vi "V7310.RTC.Get.vi"(6 "timeout ms (5000)":i32=5000, 8 "error in":errorcluster, 11 "Connection in":refnum<k5>) -> (0 "error out":errorcluster, 1 "RTC string":string, 2 "RTC":timestamp, 3 "Connection out":refnum<k5>)   [LabVIEW 2016]
uses:
  LowLevel/V7310.Commands.ctl
  <vilib>/Utility/miscctls.llb/LVDateTimeRec.ctl
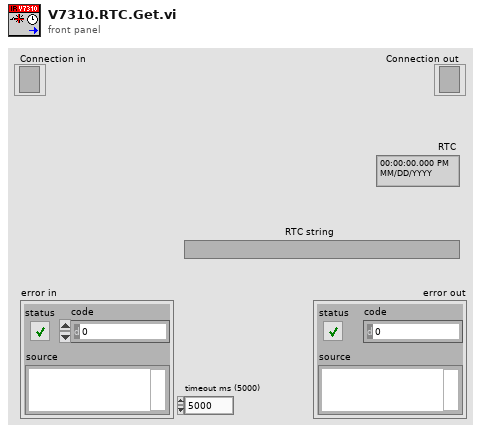
[diagram p1: front panel]
types:
  T1 = typedef "LVDateTimeRec.ctl" = cluster{"fractional second":dbl, "second":i32, "minute":i32, "hour":i32, "day of month":i32, "month":i32, "year":i32, "day of week":i32, "day of year":i32, "DST":i32}
  T2 = typedef "V7310.Commands.ctl" = enum16{"Start", "Stop", "GetStatus", "GetVarNames", "GetJobNames", "SetJob", "GetJob", "SetVars", "GetVars", "SetLayoutPosition", "SetRotation", "GetMessageID", "GetMessages", "ConfirmMessages", "DeleteMessages", "SetRTC", "GetRTC", "SetVarPosition", "SetIntensity", "GetIntensity", "SetStartTriggerDelay", "GetStartTriggerDelay", "SetStopTriggerDelay", "GetStopTriggerDelay", "SetConsecutiveTriggerDelay", "GetConsecutiveTriggerDelay", "SetMarkSpeed", "GetMarkSpeed"}
  T3 = typedef "V7310.ErrorLevels.ctl" = enum16{"OK", "Warning", "Error"}
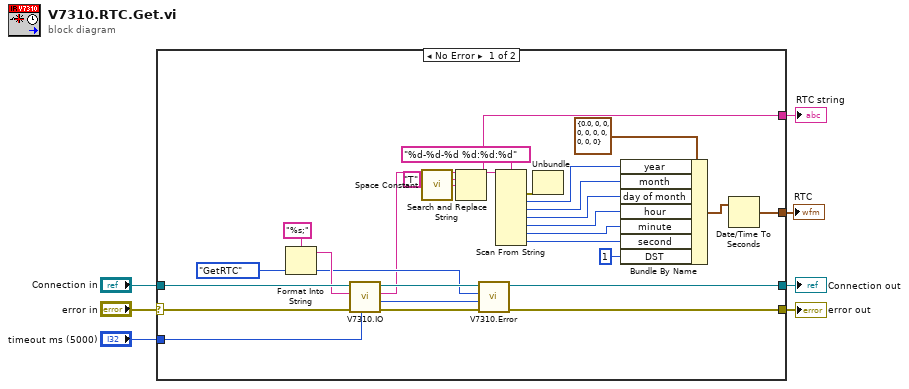
[diagram p0: block diagram]
diagram:
  n1 = case shown="No Error" "error in" {
    selector: "error in" -> [w31 w34]
    tunnel: "Connection in" -> [w32 w35]
    tunnel: [w33 w35] -> w6
    tunnel: "timeout ms (5000)" -> [w30 _]
    tunnel: [w24 w34] -> w3
    tunnel: [w23 _] -> w2
    tunnel: [w10 _] -> w1
    frame No Error {
      w27 = V7310.Commands."GetRTC" ("Cmd")
      n2 = Format Into String(format string="%s;", w27) -> (resulting string=w28:string)  [unwired: 2 in, 1 out]
      n3 = call "V7310.IO.vi"("timeout ms (5000)"=w30, "error in"=w31, "Data in"=w28, "Connection in"=w32) -> ("error out"=w25:errorcluster, "Error Level"=w26:T3, "Data out"=w20:string, "Connection out"=w33:refnum<k5>)  [unwired: 4 in]
      n4 = call <vilib>:"Space Constant.vi"() -> ("String"=w22:string)
      n5 = Search and Replace String(input string=w20, search string="T", replace string=w22) -> (result string=w10:string)  [unwired: 5 in, 3 out]
      n6 = call "V7310.Error.vi"("error in"=w25, "Error Level"=w26, "Cmd"=w27) -> ("error out"=w24:errorcluster)  [unwired: 8 in]
      n7 = Scan From String(format string="%d-%d-%d %d:%d:%d", input string=w10) -> (error out=w9:errorcluster, output 1=w17:i32, output 2=w16:i32, output 3=w15:i32, output 4=w14:i32, output 5=w13:i32, output 6=w12:i32)  [unwired: 8 in, 2 out]
      n8 = Unbundle(w9) -> ()  [unwired: 3 out]
      n9 = Bundle By Name(cluster=T1 {"fractional second"=0.0, "second"=0, "minute"=0, "hour"=0, "day of month"=0, "month"=0, "year"=0, "day of week"=0, "day of year"=0, "DST"=0} ("date time rec"), "year"=w17, "month"=w16, "day of month"=w15, "hour"=w14, "minute"=w13, "second"=w12, "DST"=1) -> (w11:T1)
      n10 = Date/Time To Seconds(2:w11) -> (0:w23:timestamp)  [unwired: 1 in]
    }
    frame Error {
    }
  }
  "Connection out" <- w6
  "error out" <- w3
  "RTC" <- w2
  "RTC string" <- w1
